vi "Does line exist.vi"(2 "Line to look for":tag, 3 "Line type":T1(ring)) -> (0 "Does line exist?":bool, 1 "Lines":tag[](array[tag]))   [LabVIEW 2015]
doc: "Returns a list of all the DAQmx lines of a given type, and whether the specified line exists in the list or not.\n\nMay be kinda slow if you have a lot of lines."
uses:
  <resource>/objmgr/daqmx.rc
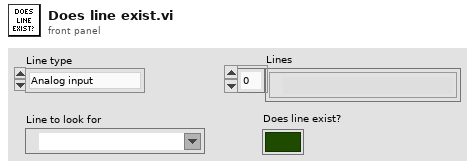
[diagram p1: front panel]
types:
  T1 = enum16{"Analog input", "Analog output", "Digital input", "Digital output", "Counter input", "Counter output"}
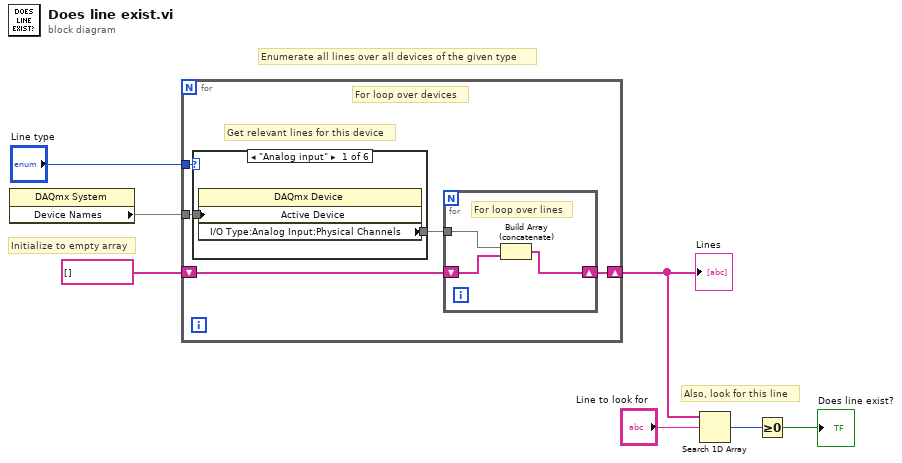
[diagram p0: block diagram]
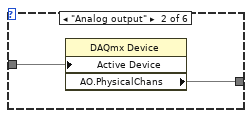
[diagram p2: hidden frame]
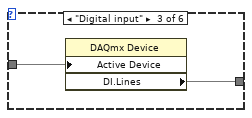
[diagram p3: hidden frame]
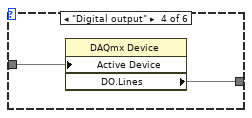
[diagram p4: hidden frame]
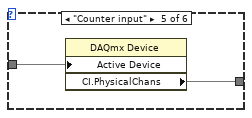
[diagram p5: hidden frame]
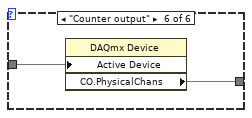
[diagram p6: hidden frame]
diagram:
  # "Also, look for this line"
  # "Initialize to empty array"
  # "Enumerate all lines over all devices of the given type"
  n1 = property class="DAQmx System"() -> ("Device Names"=w7)  [unwired: 2 in, 2 out]
  n2 = for {
    tunnel: w7 -> [w12]
    tunnel: "Line type" -> [w11]
    shift-right: [w9] -> w3
    shift-left: tag[] [] -> [w8]
    # "Get relevant lines for this device"
    # "For loop over devices"
    n3 = case shown="\"Analog input\"" w11 {
      tunnel: w12 -> [w17 w19 w21 w23 w25 w27]
      tunnel: [w16 w18 w20 w22 w24 w26] -> w10
      frame "Analog input" {
        n4 = property class="DAQmx Device"("Active Device"=w17) -> ("I/O Type:Analog Input:Physical Channels"=w16)  [unwired: 2 in, 2 out]
      }
      frame "Analog output" {
        n5 = property class="DAQmx Device"("Active Device"=w19) -> ("AO.PhysicalChans"=w18)  [unwired: 2 in, 2 out]
      }
      frame "Digital input" {
        n6 = property class="DAQmx Device"("Active Device"=w21) -> ("DI.Lines"=w20)  [unwired: 2 in, 2 out]
      }
      frame "Digital output" {
        n7 = property class="DAQmx Device"("Active Device"=w23) -> ("DO.Lines"=w22)  [unwired: 2 in, 2 out]
      }
      frame "Counter input" {
        n8 = property class="DAQmx Device"("Active Device"=w25) -> ("CI.PhysicalChans"=w24)  [unwired: 2 in, 2 out]
      }
      frame "Counter output" {
        n9 = property class="DAQmx Device"("Active Device"=w27) -> ("CO.PhysicalChans"=w26)  [unwired: 2 in, 2 out]
      }
    }
    n10 = for {
      tunnel: w10 -> [w15]
      shift-right: [w14] -> w9
      shift-left: w8 -> [w13]
      # "For loop over lines"
      n11 = Build Array (concatenate)(w15, w13) -> (w14:tag[])
    }
  }
  "Lines" <- w3
  n12 = Search 1D Array(1D array=w3, element="Line to look for") -> (index of element=w2:i32)  [unwired: 1 in]
  n13 = Greater Or Equal To 0?(x=w2) -> (x >= 0?=→"Does line exist?":bool)
